vi "5492_DriveOrientation.vi"() -> ()   [LabVIEW 2016]
panel:
  in  "Numeric":dbl
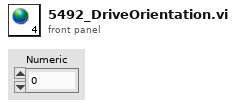
[diagram p1: front panel]
diagram:
